vi "Merge Data.vi"(8 "error in":errorcluster, 10 "Analyzed":refnum<class "Instrument.lvclass">, 11 "Acquired":refnum<class "Instrument.lvclass">) -> (0 "error out":errorcluster, 3 "Instrument out":refnum<class "Instrument.lvclass">)   [LabVIEW 2014, in "Instrument.lvclass"]
uses:
  Instrument.lvclass
  state.ctl
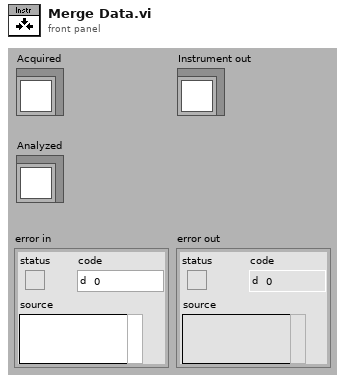
[diagram p1: front panel]
types:
  T1 = typedef "Instrument.lvclass/state.ctl" = enum8{"Configure", "Acquire", "Wait", "Quit", "Handle Error", "NOOP"}
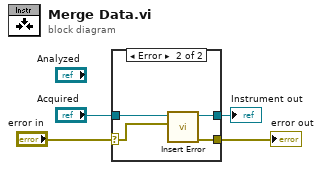
[diagram p0: block diagram]
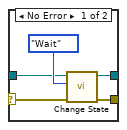
[diagram p2: hidden frame]
diagram:
  n1 = case shown="Error" "error in" {
    selector: "error in" -> [w5 w11]
    tunnel: [w8 w10] -> w3
    tunnel: [w7 w12] -> w1
    tunnel: "Acquired" -> [w6 w13]
    frame No Error {
      n2 = call "Change State.vi"("error in"=w5, "instr state"=state."Wait", "Instrument in"=w6) -> ("error out"=w8:errorcluster, "Instrument out"=w7:refnum<class "Instrument.lvclass">)  [unwired: 7 in]
    }
    frame Error {
      n3 = call "Insert Error.vi"("err"=w11, "Instrument in"=w13) -> ("error out"=w10:errorcluster, "Instrument out"=w12:refnum<class "Instrument.lvclass">)  [unwired: 7 in, 1 out]
    }
  }
  "error out" <- w3
  "Instrument out" <- w1
